vi "GetText.vi"(8 "error in":errorcluster, 11 "Temperature Chamber Model editor node in":refnum<class "Temperature Chamber Model editor node.lvclass">) -> (0 "error out":errorcluster, 1 "additional text":string, 2 "text":string, 3 "Temperature Chamber Model editor node out":refnum<class "Temperature Chamber Model editor node.lvclass">, 4 "glyph":string)   [LabVIEW 2013, in "Temperature Chamber Model editor node.lvclass"]
uses:
  Temperature Chamber Model editor node.lvclass
  <vilib>/NI/DCAF/Tag Editor Core/control module/editor node/control module editor.lvclass
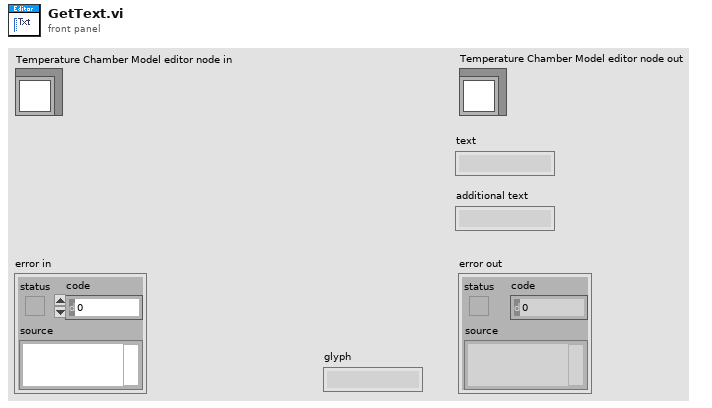
[diagram p1: front panel]
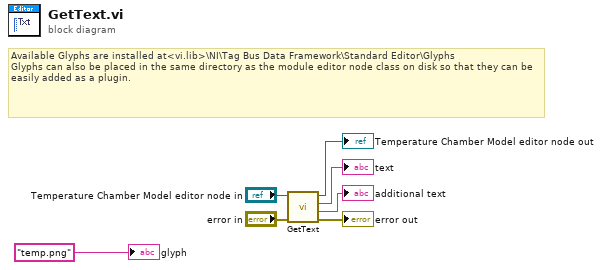
[diagram p0: block diagram]
diagram:
  # "Available Glyphs are installed at<vi.lib>\\NI\\Tag Bus Data Framework\\Standard Editor\\Glyphs\nGlyphs can also be placed in the same directory as the module editor node class on disk so that they can be easily added as a plugin."
  n1 = call-parent "GetText.vi"("error in"="error in", "Module Editor Node in"="Temperature Chamber Model editor node in") -> ("error out"=→"error out":errorcluster, "additional text"=→"additional text":string, "text"=→"text":string, "Module Editor Node out"=→"Temperature Chamber Model editor node out":refnum<class "Temperature Chamber Model editor node.lvclass">)  [unwired: 5 in, 1 out]
  "glyph" <- "temp.png" ("glyph")
